vi "SetControls.vi"(1 "Controls":refnum<vi>[](array[refnum]), 2 "Enable?":bool) -> ()   [LabVIEW 2012]
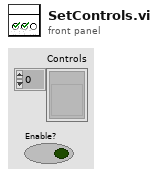
[diagram p1: front panel]
types:
  T1 = enum8{"Enabled", "Disabled", "Disabled and Grayed Out"}
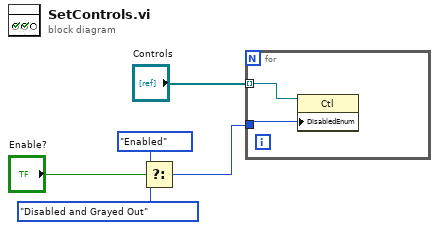
[diagram p0: block diagram]
diagram:
  n1 = Select(t=T1."Enabled" ("Disabled"), s="Enable?", f=T1."Disabled and Grayed Out" ("Disabled")) -> (s? t:f=w4:T1)
  n2 = for {
    tunnel: "Controls" -> [w7] mode=indexing
    tunnel: w4 -> [w6]
    n3 = property class="Ctl"(reference=w7, "DisabledEnum"=w6) -> ()  [unwired: 1 in, 2 out]
  }
